vi "ziModFinish.vi"(7 "Error In":errorcluster, 10 "ziModHandle In":T1 {"ModHandle" format="0x%08x"; "Conn" format="0x%08x"}) -> (0 "Error Out":errorcluster, 3 "ziModHandle Out":T1 {"ModHandle" format="0x%08x"; "Conn" format="0x%08x"})   [LabVIEW 2018, in "Zurich Instruments LabOne.lvlib"]
doc: "Stops a running module but does not destroy it."
uses:
  Zurich Instruments LabOne.lvlib
  <instrlib>/Zurich Instruments LabOne/Private/ziLV64.framework
  ziTypeModHandle.ctl
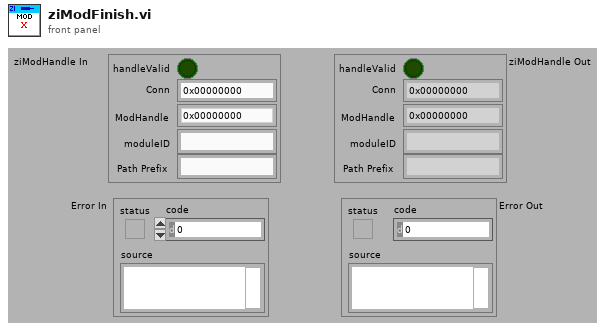
[diagram p1: front panel]
types:
  T1 = typedef "Zurich Instruments LabOne.lvlib/ziTypeModHandle.ctl" = cluster{"handleValid":bool, "Conn":u64, "ModHandle":u64, "moduleID":string, "Path Prefix":string}
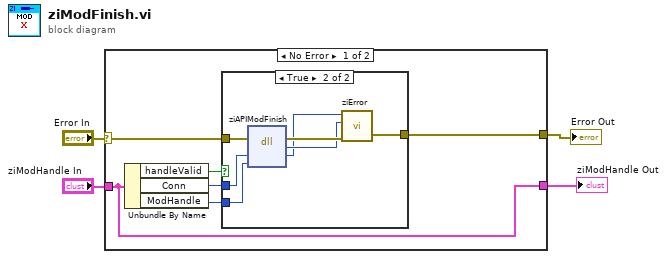
[diagram p0: block diagram]
diagram:
  n1 = case shown="No Error" "Error In" {
    selector: "Error In" -> [w9 w20]
    tunnel: "ziModHandle In" -> [w5 w19]
    tunnel: [w10 w20] -> w4
    tunnel: [w5 w19] -> w1
    frame No Error {
      n2 = Unbundle By Name(w5) -> ("handleValid"=w8:bool, "Conn"=w7:u64, "ModHandle"=w6:u64)
      n3 = case shown="True" w8 {
        tunnel: w9 -> [w11 w18]
        tunnel: [w11 w15] -> w10
        tunnel: w7 -> [_ w14]
        tunnel: w6 -> [_ w13]
        frame False {
        }
        frame True {
          n4 = dll-call lib="Applications/National Instruments/LabVIEW 2019 64-bit/instr.lib/Zurich Instruments LabOne/Private/ziLV*.*" fn="ziAPIModFinish"(error in=w18, "conn"=w14, "ModHandle"=w13) -> (error out=w17:errorcluster, "return type"=w16:u32, "conn"=w12:u64)  [unwired: 3 in, 1 out]
          n5 = call "ziError.vi"("Conn"=w12, "ziErrorCode"=w16, "Error In"=w17) -> ("Error Out"=w15:errorcluster)  [unwired: 2 in, 1 out]
        }
      }
    }
    frame Error {
    }
  }
  "Error Out" <- w4
  "ziModHandle Out" <- w1
